vi "Log_FGV.vi"(11 "Limit of logs":i32) -> (3 "List of logs":string)   [LabVIEW 2020]
uses:
  #typedef_LogsAction.ctl
  #typedef_Log.ctl
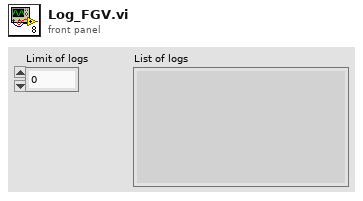
[diagram p1: front panel]
types:
  T1 = typedef "#typedef_Log.ctl" = cluster{"Info":string, "Time and data of log's registration":timestamp}
  T2 = typedef "#typedef_LogsAction.ctl" = enum16{"ClearList", "AddRecord", "GetList"}
  T3 = typedef "LVDateTimeRec.ctl" = cluster{"fractional second":dbl, "second":i32, "minute":i32, "hour":i32, "day of month":i32, "month":i32, "year":i32, "day of week":i32, "day of year":i32, "DST":i32}
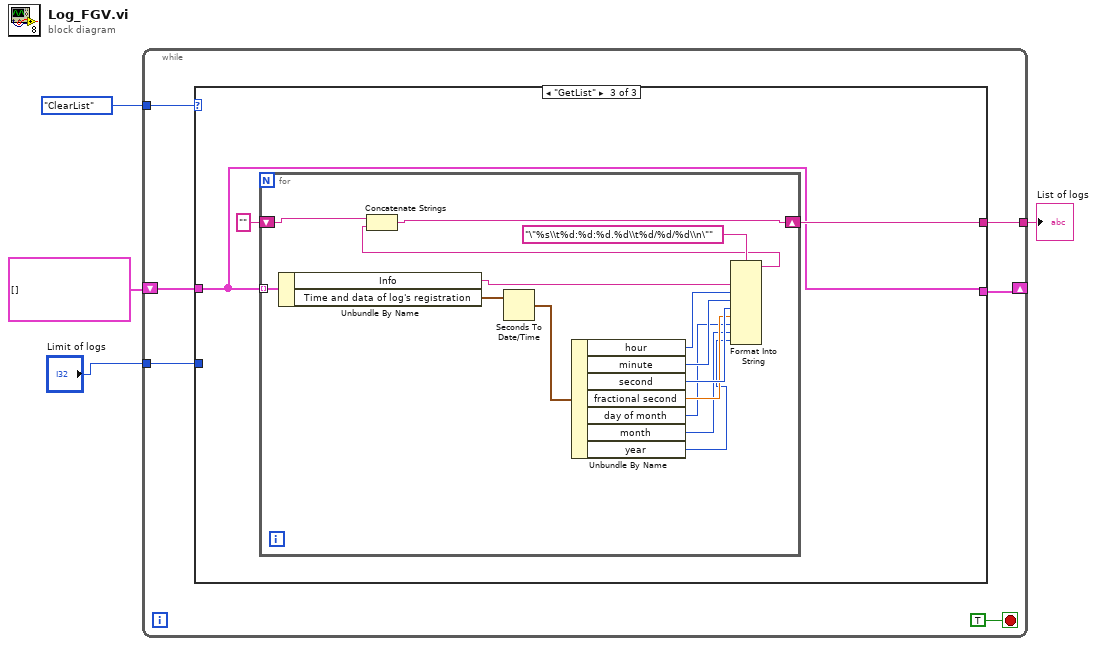
[diagram p0: block diagram]
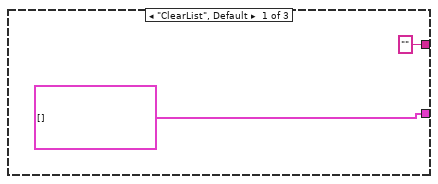
[diagram p2: hidden frame]
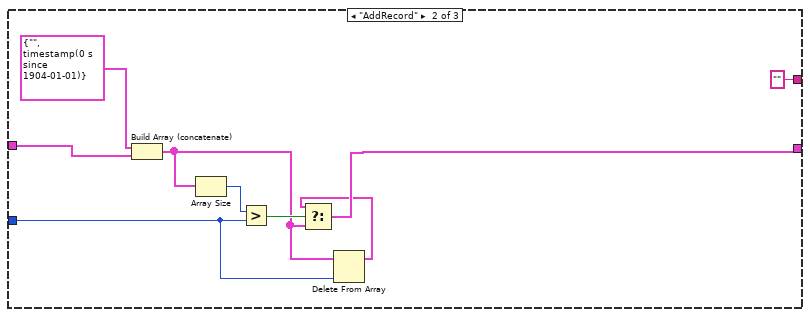
[diagram p3: hidden frame]
diagram:
  n1 = while {
    tunnel: #typedef_LogsAction."ClearList" ("Action") -> [w9]
    shift-right: [w7] -> _
    shift-left: T1[] [] -> [w8]
    tunnel: "Limit of logs" -> [w6]
    tunnel: [w5] -> w4
    stop <- TRUE stop-if-true
    n2 = case shown="\"GetList\"" w9 {
      tunnel: w8 -> [_ w20 w23]
      tunnel: [T1[] [] w18 w23] -> w7
      tunnel: w6 -> [_ w14 _]
      tunnel: ["" "" w24] -> w5
      frame "ClearList", Default {
      }
      frame "AddRecord" {
        n3 = Build Array (concatenate)(T1 {"Info"="", "Time and data of log's registration"=timestamp(0 s since 1904-01-01)} ("Logs"), w20) -> (w17:T1[])
        n4 = Array Size(array=w17) -> (size(s)=w16:i32)
        n5 = Greater?(x=w16, y=w14) -> (0:w19:bool)
        n6 = Delete From Array(array=w17, index=w14) -> (array with subset deleted=w15:T1[])  [unwired: 1 in, 1 out]
        n7 = Select(t=w15, s=w19, f=w17) -> (s? t:f=w18:T1[])
      }
      frame "GetList" {
        n8 = for {
          tunnel: w23 -> [w39] mode=indexing
          shift-right: [w25] -> w24
          shift-left: "" -> [w27]
          n9 = Unbundle By Name(w39) -> ("Info"=w36:string, "Time and data of log's registration"=w38:timestamp)
          n10 = Seconds To Date/Time(time stamp (now)=w38) -> (date time rec=w37:T3)  [unwired: 1 in]
          n11 = Unbundle By Name(w37) -> ("hour"=w34:i32, "minute"=w33:i32, "second"=w32:i32, "fractional second"=w31:dbl, "day of month"=w30:i32, "month"=w29:i32, "year"=w28:i32)
          n12 = Format Into String(format string="\"%s\\t%d:%d:%d.%d\\t%d/%d/%d\\n\"", w36, w34, w33, w32, w31, w30, w29, w28) -> (resulting string=w26:string)  [unwired: 2 in, 1 out]
          n13 = Concatenate Strings(w27, w26) -> (w25:string)
        }
      }
    }
  }
  "List of logs" <- w4
